vi "buenas noches.vi"   [LabVIEW 2016]
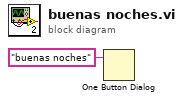
[diagram p0: block diagram]
diagram:
  n1 = One Button Dialog(message="buenas noches") -> ()  [unwired: 1 in, 1 out]
